vi "SetVoltage.vi"(8 "error in":errorcluster, 10 "Input Voltage":dbl min=0.0 max=100.0 step=0.1, 11 "VISA Ket":refnum<visa-resource-name>) -> (0 "error out":errorcluster, 3 "VISA Ket":refnum<visa-resource-name>)   [LabVIEW 2012]
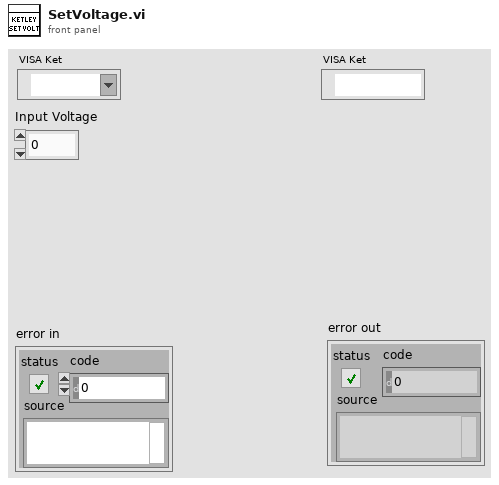
[diagram p1: front panel]
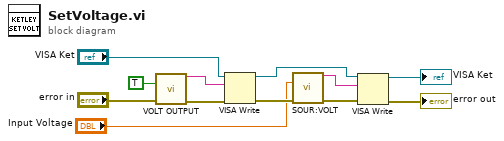
[diagram p0: block diagram]
diagram:
  n1 = call "VOLT OUTPUT"("VOLTOUTPUT"=TRUE ("On?"), "error in (no error)"="error in") -> ("Result"=w1:string, "error out"=w5:errorcluster)  [unwired: 12 in]
  n2 = VISA Write(VISA resource name="VISA Ket", write buffer=w1, error in (no error)=w5) -> (VISA resource name out=w6:refnum<visa-resource-name>, error out=w7:errorcluster)  [unwired: 1 out]
  n3 = call "SOUR:VOLT"("VOLT"="Input Voltage", "error in (no error)"=w7) -> ("Result"=w10:string, "error out"=w11:errorcluster)  [unwired: 12 in]
  n4 = VISA Write(VISA resource name=w6, write buffer=w10, error in (no error)=w11) -> (VISA resource name out=→"VISA Ket":refnum<visa-resource-name>, error out=→"error out":errorcluster)  [unwired: 1 out]
